vi "RobotPoseEstimator.vi"(9 "real x y theta (k)":cluster{"xr":dbl, "yr":dbl, "thetar":dbl}, 10 "NL":dbl, 11 "NR":dbl) -> (0 "real v and w":cluster{"vr":dbl, "wr":dbl}, 8 "real x y theta (k+1)":cluster{"xr+1":dbl, "yr+1":dbl, "thetar+1":dbl} {"thetar+1" format="%#_6f"; "yr+1" format="%#_6f"; "xr+1" format="%#_6f"})   [LabVIEW 2016]
panel:
  in  "deltat":dbl=0.15
  in  "l":dbl=0.365
  in  "r":dbl=0.046
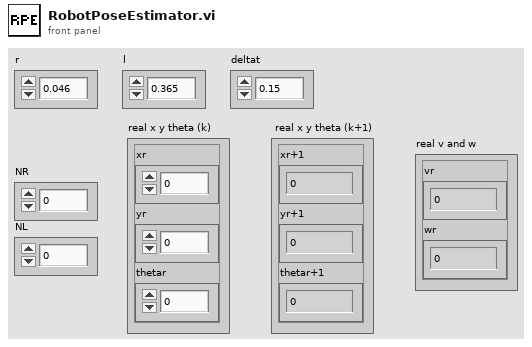
[diagram p1: front panel]
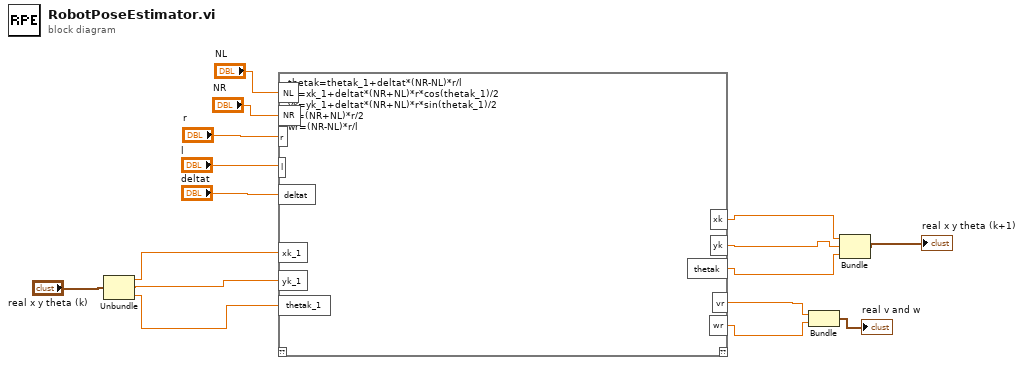
[diagram p0: block diagram]
diagram:
  n1 = Unbundle("real x y theta (k)") -> ("xr"=w10:dbl, "yr"=w9:dbl, "thetar"=w8:dbl)
  n2 = script code="thetak=thetak_1+deltat*(NR-NL)*r/l\nxk=xk_1+deltat*(NR+NL)*r*cos(thetak_1)/2\nyk=yk_1+deltat*(NR+NL)*r*sin(thetak_1)/2\nvr=(NR+NL)*r/2\nwr=(NR-NL)*r/l"("r"="r", "l"="l", "deltat"="deltat", "xk_1"=w10, "yk_1"=w9, "thetak_1"=w8, "NL"="NL", "NR"="NR") -> ("xk"=w6:dbl, "yk"=w5:dbl, "thetak"=w4:dbl, "vr"=w3:dbl, "wr"=w2:dbl)  [unwired: 1 in, 1 out]
  n3 = Bundle(w3, w2) -> (→"real v and w":cluster{dbl, dbl})  [unwired: 1 in]
  n4 = Bundle(w6, w5, w4) -> (→"real x y theta (k+1)":cluster{dbl, dbl, dbl})  [unwired: 1 in]
